vi "MoveCartesian.vi"(0 "error in (no error)":errorcluster, 1 "HighSpeedEServer":refnum<k24>, 2 "Pose":T1, 3 "Speed":cluster{"classification":i32, "speed":dbl} {"classification" items=["LinkPercent", "Cartesian_MM_S", "Cartesian_DEG_S"]}, 4 "Coordinate":cluster{"userCoordinate":i32, "coordinate":i32}={"userCoordinate"=0, "coordinate"=16} {"coordinate" items=["Base"=16, "Robot"=17, "User"=18, "Tool"=19]}, 5 "tool":i32, 6 "RCONF":i32, 7 "commandtype":i32(ring)=1 items=["LinkAbsolute"=1, "StraightAbsolute"=2, "StraightIncrement"=3]) -> (20 "error out":errorcluster)   [LabVIEW 2023, in "UnderAutomation.Yaskawa.lvlib"]
uses:
  UnderAutomation.Yaskawa.lvlib
  C:/Users/fg/Documents/Yaskawa.vi/LabVIEW_2024/UnderAutomation.Yaskawa/lib/UnderAutomation.Yaskawa.dll
  LabVIEW_2024/UnderAutomation.Yaskawa/lib/UnderAutomation.Yaskawa.dll
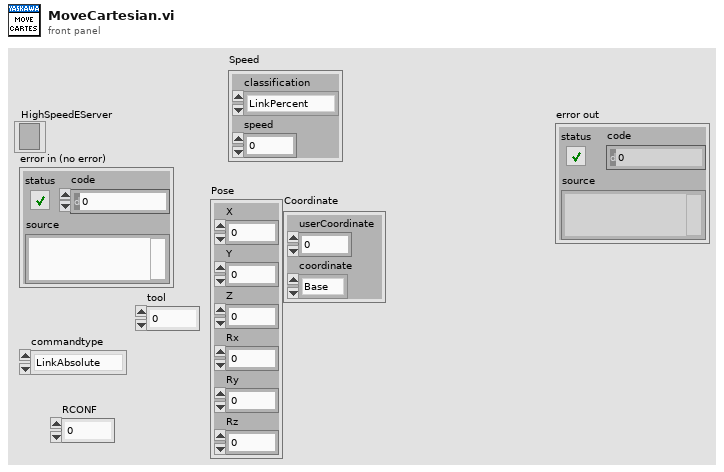
[diagram p1: front panel]
types:
  T1 = cluster{"X":dbl, "Y":dbl, "Z":dbl, "Rx":dbl, "Ry":dbl, "Rz":dbl}
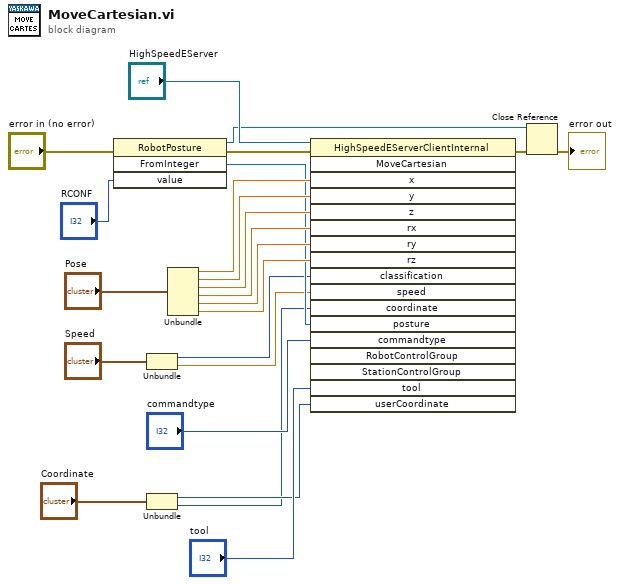
[diagram p0: block diagram]
diagram:
  n1 = invoke class="RobotPosture" method="FromInteger"(error in="error in (no error)", "value"="RCONF") -> (reference out=w1:refnum<k24>, error out=w10:errorcluster, "FromInteger"=w13:refnum<k24>)  [unwired: 2 in, 1 out]
  n2 = Unbundle("Speed") -> ("classification"=w8:i32, "speed"=w7:dbl)
  n3 = Unbundle("Coordinate") -> ("userCoordinate"=w5:i32, "coordinate"=w4:i32)
  n4 = Unbundle("Pose") -> ("X"=w21:dbl, "Y"=w20:dbl, "Z"=w19:dbl, "Rx"=w18:dbl, "Ry"=w17:dbl, "Rz"=w16:dbl)
  n5 = invoke class="HighSpeedEServerClientInternal" method="MoveCartesian"(reference="HighSpeedEServer", error in=w10, "x"=w21, "y"=w20, "z"=w19, "rx"=w18, "ry"=w17, "rz"=w16, "classification"=w8, "speed"=w7, "coordinate"=w4, "posture"=w13, "commandtype"="commandtype", "tool"="tool", "userCoordinate"=w5) -> (error out=w3:errorcluster)  [unwired: 3 in, 17 out]
  n6 = Close Reference(reference=w1, error in (no error)=w3) -> (error out=→"error out":errorcluster)
